vi "subCalculate_SetScaleBar.vi"(5 "ROI in":T2={"Bin"=2, "ROI"={"x offset"=256, "y offset"=256, "x width"=512, "y width"=512}} caption="ROI" {"ROI"."x offset" min=1 max=512 step=1; "ROI"."y offset" min=1 max=512 step=1; "ROI"."x width" min=1 max=512 step=1; "ROI"."y width" min=1 max=512 step=1; "Bin" items=["1x1"=1, "2x2"=2, "4x4"=4]}, 6 "Scale calculation cluster":T1, 7 "TI-Ctrl":T3={"Obj"=2, "Cube Bottom"=1, "Cube Top"=1, "PFS-Ctrl"={"PFS IO"=FALSE, "PSF Err"=FALSE, "PSF Pos"=0}, "Z-Ctrl"={"Z-pos"=500.175, "Home"=FALSE, "Sensitivity"=1}, "Condenser"=1, "Lightpath"=enum."EYE"} {"Condenser" items=["A"=1, "DICN2"=2, "- empty 3 -"=3, "- empty 4 -"=4, "- empty 5 -"=5, "- empty 6 -"=6]; "Z-Ctrl"."Sensitivity" min=1 max=3 step=1 scale=1.0..3.0; "PFS-Ctrl"."PSF Pos" scale=0.0..16400.0; "Cube Top" items=["Cy5"=1, "RFP"=2, "DM532"=3, "DM488"=4, "DM405"=5, "- empty 6 -"=6]; "Cube Bottom" items=["405/488/532/642"=1, "- empty 2 -"=2, "EM585/65"=3, "EM525/50"=4, "EM460/50"=5, "DIC"=6]; "Obj" items=["20x/.75 Dry PFS"=1, "40x/1.3 Oil PFS"=2, "60x/1.4 Oil PFS"=3, "- empty 4 -"=4, "- empty 5 -"=5, "- empty 6 -"=6]}, 8 "error in":errorcluster, 11 "Handle in":u32) -> (0 "error out":errorcluster, 3 "Handle out":u32)   [LabVIEW 2015]
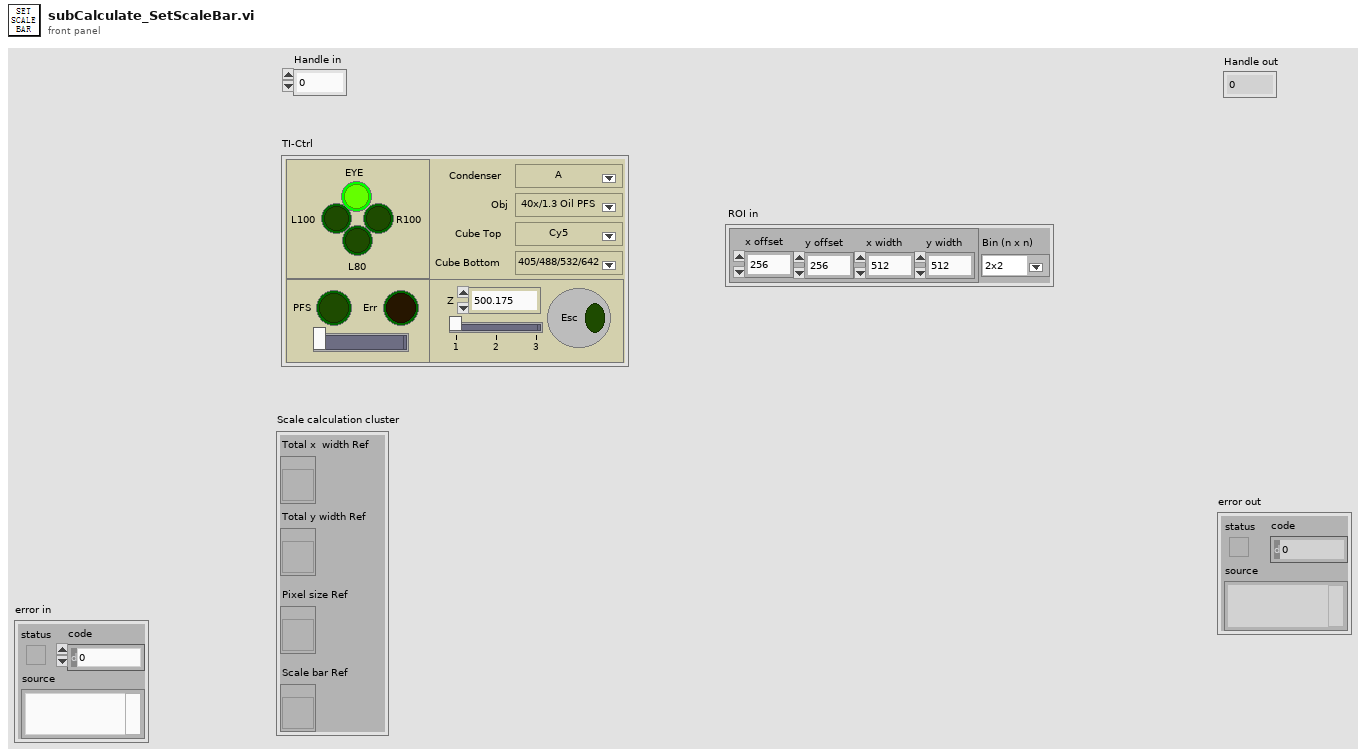
[diagram p1: front panel]
types:
  T1 = cluster{"Total x  width Ref":refnum<vi>, "Total y width Ref":refnum<vi>, "Pixel size Ref":refnum<vi>, "Scale bar Ref":refnum<vi>}
  T2 = cluster{"Bin":u16, "ROI":cluster{"x offset":i32, "y offset":i32, "x width":i32, "y width":i32}}
  T3 = cluster{"Obj":u16, "Cube Bottom":u16, "Cube Top":u16, "PFS-Ctrl":cluster{"PFS IO":bool, "PSF Err":bool, "PSF Pos":u32}, "Z-Ctrl":cluster{"Z-pos":dbl, "Home":bool, "Sensitivity":u8}, "Condenser":u16, "Lightpath":enum32{"EYE", "L100", "R100", "L80"}}
  T4 = enum8{"Enabled", "Disabled", "Disabled and Grayed Out"}
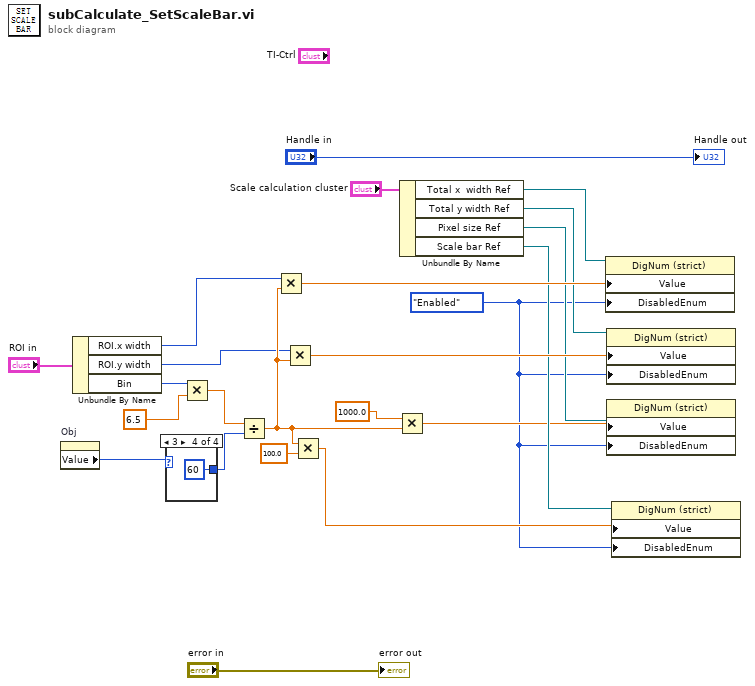
[diagram p0: block diagram]
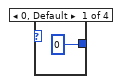
[diagram p2: hidden frame]
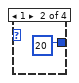
[diagram p3: hidden frame]
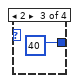
[diagram p4: hidden frame]
diagram:
  w2 = T4."Enabled" ("Disabled")
  n1 = property on="Obj" class="Ring (strict)"() -> ("Value"=w13:u16)  [unwired: 2 in, 2 out]
  n2 = Unbundle By Name("ROI in") -> ("ROI.x width"=w14:i32, "ROI.y width"=w15:i32, "Bin"=w17:u16)
  n3 = case shown="3" w13 {
    tunnel: [0 20 40 60] -> w20
    frame 0, Default {
    }
    frame 1 {
    }
    frame 2 {
    }
    frame 3 {
    }
  }
  n4 = Multiply(x=w17, y=6.5) -> (x*y=w21:dbl)
  n5 = Divide(x=w21, y=w20) -> (x/y=w16:dbl)
  n6 = Multiply(x=w14, y=w16) -> (x*y=w9:dbl)
  n7 = Multiply(x=w15, y=w16) -> (x*y=w7:dbl)
  n8 = Multiply(x=w16, y=100.0) -> (x*y=w4:dbl)
  n9 = Multiply(x=1000.0, y=w16) -> (x*y=w3:dbl)
  n10 = Unbundle By Name("Scale calculation cluster") -> ("Total x  width Ref"=w10:refnum<vi>, "Total y width Ref"=w8:refnum<vi>, "Pixel size Ref"=w6:refnum<vi>, "Scale bar Ref"=w5:refnum<vi>)
  n11 = property class="DigNum (strict)"(reference=w10, "Value"=w9, "DisabledEnum"=w2) -> ()  [unwired: 1 in, 2 out]
  n12 = property class="DigNum (strict)"(reference=w8, "Value"=w7, "DisabledEnum"=w2) -> ()  [unwired: 1 in, 2 out]
  n13 = property class="DigNum (strict)"(reference=w6, "Value"=w3, "DisabledEnum"=w2) -> ()  [unwired: 1 in, 2 out]
  n14 = property class="DigNum (strict)"(reference=w5, "Value"=w4, "DisabledEnum"=w2) -> ()  [unwired: 1 in, 2 out]
  "error out" <- "error in"
  "Handle out" <- "Handle in"
